vi "datadecoder.vi"(6 "error in":errorcluster, 7 "FPGA VI Reference Out":refnum<k20>) -> ()   [LabVIEW 2012]
uses:
  RIOGlobal.vi
  <vilib>/Utility/error.llb/Error Cluster From Error Code.vi
  <vilib>/rvi/errors/niLvFpgaAdjustHostInterfaceError.vi
  <vilib>/rvi/interface/nirviReadWriteControl/nirviReadWriteControl.xnode
  NiFpgaLv.dll
  <vilib>/rvi/interface/Simulation/niFpgaSimulationCallBeginRW.vi
  <vilib>/ptbypt/NI_PtbyPt.lvlib
panel:
  out "error out 2":errorcluster
  out "Auto":bool
  out "Run":bool
  out "E - STOP":bool
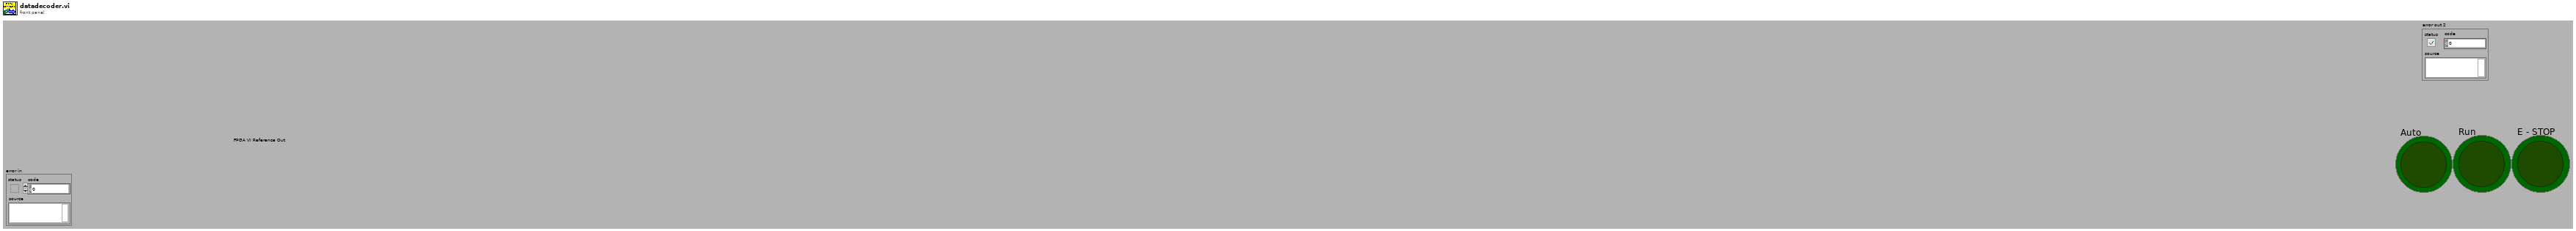
[diagram p1: front panel]
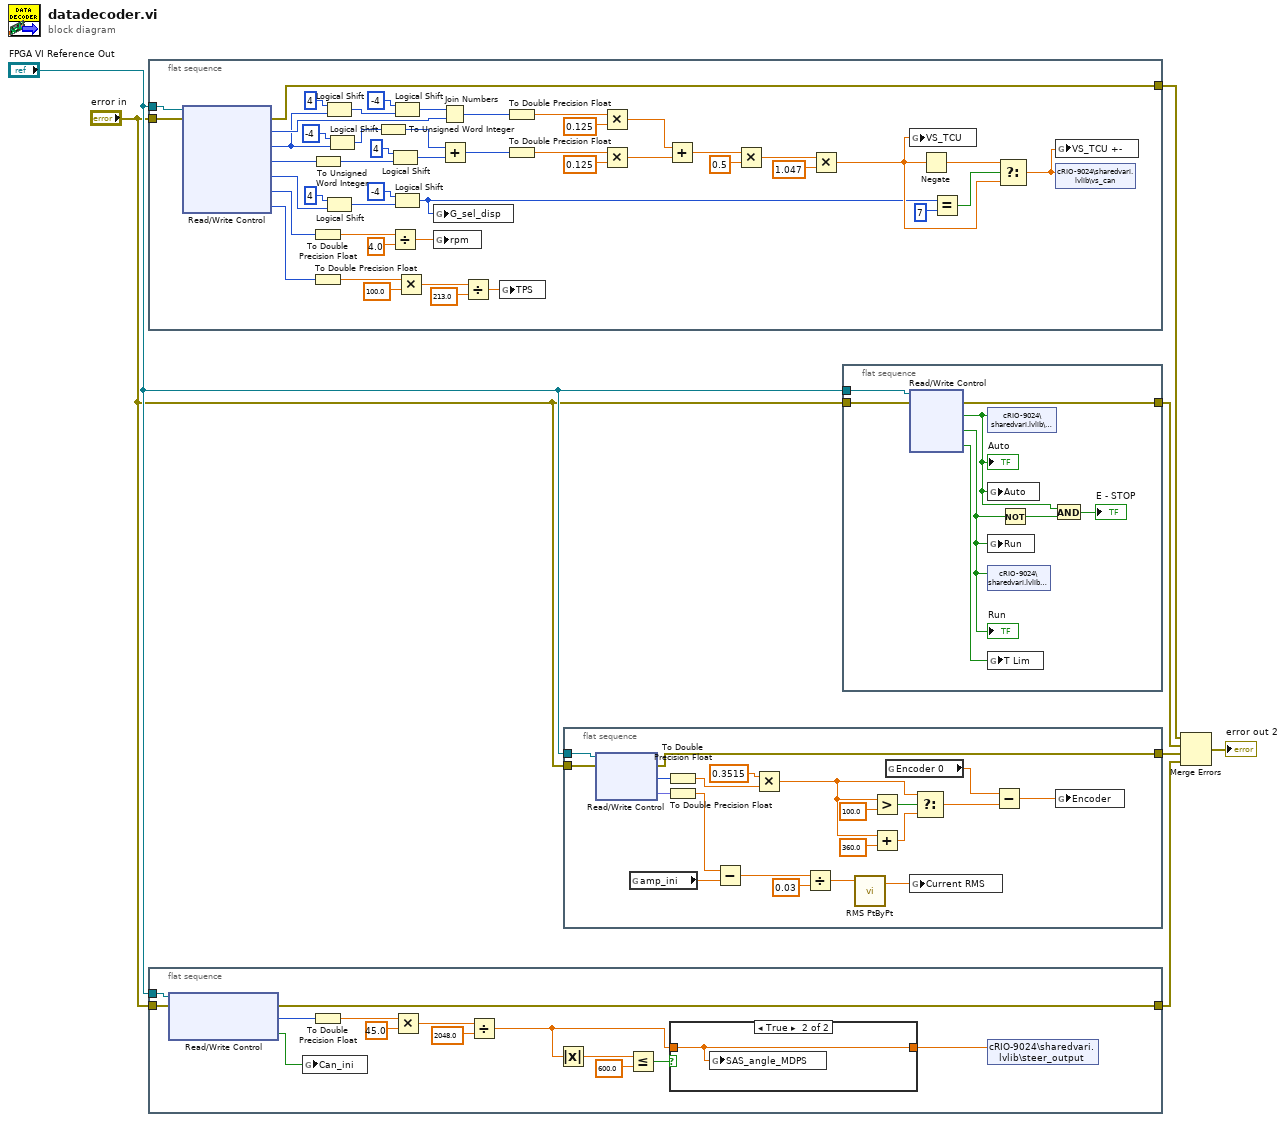
[diagram p0: block diagram]
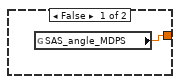
[diagram p2: hidden frame]
diagram:
  n1 = flat-sequence {
    tunnel: "FPGA VI Reference Out" -> [w55]
    tunnel: "error in" -> [w54]
    tunnel: [w8] -> w5
    frame #0 {
      n2 = xnode "Read/Write Control"("FPGA VI Reference In"=w55, "error in"=w54) -> ("error out"=w8:errorcluster, "WHEEL_RL"=w51:u8, "WHEEL_RRRL"=w42:u8, "WHELL_RR"=w41:u8, "G_sel_disp"=w21:u8, "rpm"=w11:u16, "TPS"=w10:u8)  [unwired: 1 out]
      n3 = To Unsigned Word Integer(number=w41) -> (unsigned 16bit integer=w40:u16)
      n4 = To Double Precision Float(number=w11) -> (double precision float=w19:dbl)
      n5 = To Double Precision Float(number=w10) -> (double precision float=w15:dbl)
      n6 = Logical Shift(y=i16 4, x=w42) -> (x << y=w43:u8)
      n7 = Logical Shift(y=i16 4, x=w21) -> (x << y=w23:u8)
      n8 = Logical Shift(y=i16 -4, x=w42) -> (x << y=w36:u8)
      n9 = To Unsigned Word Integer(number=w36) -> (unsigned 16bit integer=w35:u16)
      n10 = Logical Shift(y=i8 4, x=w40) -> (x << y=w38:u16)
      n11 = Divide(x=w19, y=4.0) -> (x/y=w17:dbl)
      n12 = Logical Shift(y=i16 -4, x=w43) -> (x << y=w50:u8)
      n13 = Logical Shift(y=i16 -4, x=w23) -> (x << y=w20:u8)
      n14 = Multiply(x=w15, y=100.0) -> (x*y=w13:dbl)
      n15 = global write "RIOGlobal.vi" "G_sel_disp"(w20) -> ()
      n16 = global write "RIOGlobal.vi" "rpm"(w17) -> ()
      n17 = Join Numbers(hi=w50, lo=w51) -> ((hi.lo)=w48:u16)
      n18 = Add(x=w35, y=w38) -> (x+y=w37:u16)
      n19 = Divide(x=w13, y=213.0) -> (x/y=w16:dbl)
      n20 = global write "RIOGlobal.vi" "TPS"(w16) -> ()
      n21 = To Double Precision Float(number=w48) -> (double precision float=w49:dbl)
      n22 = To Double Precision Float(number=w37) -> (double precision float=w45:dbl)
      n23 = Multiply(x=w49, y=0.125) -> (x*y=w33:dbl)
      n24 = Multiply(x=w45, y=0.125) -> (x*y=w32:dbl)
      n25 = Add(x=w33, y=w32) -> (x+y=w26:dbl)
      n26 = Multiply(x=w26, y=0.5) -> (x*y=w25:dbl)
      n27 = Multiply(x=w25, y=1.047) -> (x*y=w28:dbl)
      n28 = global write "RIOGlobal.vi" "VS_TCU"(w28) -> ()
      n29 = Negate(x=w28) -> (-x=w29:dbl)
      n30 = Equal?(x=w20, y=u8 7) -> (x = y?=w30:bool)
      n31 = Select(t=w29, s=w30, f=w28) -> (s? t:f=w9:dbl)
      n32 = global write "RIOGlobal.vi" "VS_TCU +-"(w9) -> ()
      n33 = shared-variable "cRIO-9024\\sharedvari.lvlib\\vs_can"(w9) -> ()  [unwired: 1 in, 1 out]
    }
  }
  n34 = flat-sequence {
    tunnel: "FPGA VI Reference Out" -> [w63]
    tunnel: "error in" -> [w64]
    tunnel: [w56] -> w2
    frame #0 {
      n35 = xnode "Read/Write Control"("FPGA VI Reference In"=w63, "error in"=w64) -> ("error out"=w56:errorcluster, "SAS_angle_MDPS"=w69:i32, "lock on"=w58:bool)  [unwired: 1 out]
      n36 = global write "RIOGlobal.vi" "Can_ini"(w58) -> ()
      n37 = To Double Precision Float(number=w69) -> (double precision float=w67:dbl)
      n38 = Multiply(x=w67, y=45.0) -> (x*y=w66:dbl)
      n39 = Divide(x=w66, y=2048.0) -> (x/y=w59:dbl)
      n40 = Absolute Value(x=w59) -> (abs(x)=w62:dbl)
      n41 = Less Or Equal?(x=w62, y=600.0) -> (x <= y?=w60:bool)
      n42 = case shown="True" w60 {
        tunnel: w59 -> [_ w71]
        tunnel: [w70 w71] -> w57
        frame False {
          n43 = global read "RIOGlobal.vi" "SAS_angle_MDPS"() -> (w70:dbl)
        }
        frame True {
          n44 = global write "RIOGlobal.vi" "SAS_angle_MDPS"(w71) -> ()
        }
      }
      n45 = shared-variable "cRIO-9024\\sharedvari.lvlib\\steer_output"(w57) -> ()  [unwired: 1 in, 1 out]
    }
  }
  n46 = flat-sequence {
    tunnel: "FPGA VI Reference Out" -> [w74]
    tunnel: "error in" -> [w73]
    tunnel: [w72] -> w3
    frame #0 {
      n47 = xnode "Read/Write Control"("FPGA VI Reference In"=w74, "error in"=w73) -> ("error out"=w72:errorcluster, "encoder"=w80:u16, "amp"=w85:fxp<+/-,16,5>)  [unwired: 1 out]
      n48 = global read "RIOGlobal.vi" "amp_ini"() -> (w88:dbl)
      n49 = To Double Precision Float(number=w80) -> (double precision float=w81:dbl)
      n50 = To Double Precision Float(number=w85) -> (double precision float=w86:dbl)
      n51 = Subtract(x=w86, y=w88) -> (x-y=w84:dbl)
      n52 = Multiply(x=0.3515 ("y"), y=w81) -> (x*y=w89:dbl)
      n53 = Divide(x=w84, y=0.03) -> (x/y=w83:dbl)
      n54 = call <vilib>:"RMS PtByPt.vi"("x"=w83) -> ("rms value"=w92:dbl)  [unwired: 3 in, 1 out]
      n55 = Greater?(x=w89, y=100.0) -> (0:w77:bool)
      n56 = Add(x=w89, y=360.0) -> (x+y=w75:dbl)
      n57 = global read "RIOGlobal.vi" "Encoder 0"() -> (w79:dbl)
      n58 = global write "RIOGlobal.vi" "Current RMS"(w92) -> ()
      n59 = Select(t=w89, s=w77, f=w75) -> (s? t:f=w91:dbl)
      n60 = Subtract(x=w79, y=w91) -> (x-y=w90:dbl)
      n61 = global write "RIOGlobal.vi" "Encoder"(w90) -> ()
    }
  }
  n62 = flat-sequence {
    tunnel: "FPGA VI Reference Out" -> [w100]
    tunnel: "error in" -> [w99]
    tunnel: [w93] -> w4
    frame #0 {
      n63 = xnode "Read/Write Control"("FPGA VI Reference In"=w100, "error in"=w99) -> ("error out"=w93:errorcluster, "Auto"=w96:bool, "Run"=w95:bool, "T Lim"=w94:bool)  [unwired: 1 out]
      "Auto" <- w96
      "Run" <- w95
      n64 = shared-variable "cRIO-9024\\sharedvari.lvlib\\auto"(w96) -> ()  [unwired: 1 in, 1 out]
      n65 = global write "RIOGlobal.vi" "Auto"(w96) -> ()
      n66 = global write "RIOGlobal.vi" "Run"(w95) -> ()
      n67 = shared-variable "cRIO-9024\\sharedvari.lvlib\\run"(w95) -> ()  [unwired: 1 in, 1 out]
      n68 = global write "RIOGlobal.vi" "T Lim"(w94) -> ()
      n69 = Not(x=w95) -> (.not. x?=w98:bool)
      n70 = And(x=w96, y=w98) -> (x .and. y?=→"E - STOP":bool)
    }
  }
  n71 = Merge Errors(w5, w4, w3, w2) -> (→"error out 2":errorcluster)
